vi "Functional Global - Raw Inputs and Outputs.vi"(7 "Functional Global Operation (Read)":T1=enum."Read", 10 "Outputs in":dbl[](array[numeric]), 11 "Inputs in":dbl[](array[numeric])) -> (2 "Outputs out":dbl[](array[numeric]), 3 "Inputs out":dbl[](array[numeric]))   [LabVIEW 2017]
uses:
  controls/Functional Global Operation.ctl
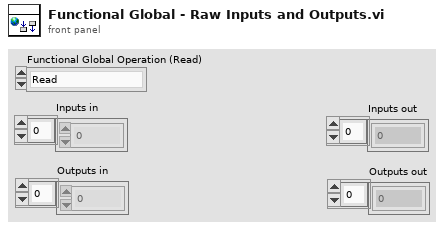
[diagram p1: front panel]
types:
  T1 = typedef "Functional Global Operation.ctl" = enum16{"Initialize", "Read", "Write"}
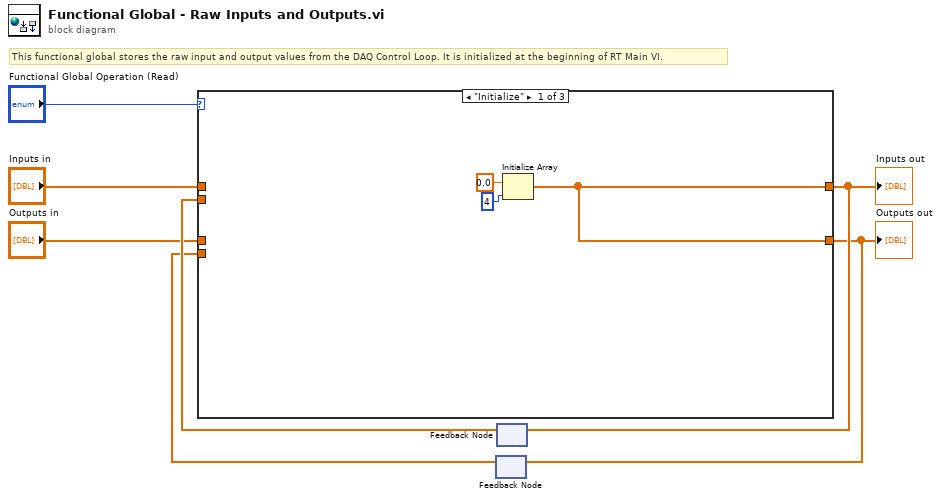
[diagram p0: block diagram]
diagram:
  # "This functional global stores the raw input and output values from the DAQ Control Loop. It is initialized at the beginning of RT Main VI."
  n1 = feedback #1() -> (w1:dbl[])  [unwired: 1 in]
  n2 = feedback #2() -> (w5:dbl[])  [unwired: 1 in]
  n3 = case shown="\"Initialize\"" "Functional Global Operation (Read)" {
    tunnel: "Inputs in" -> [_ _ w14]
    tunnel: [w8 w12 w14] -> w4
    tunnel: w5 -> [_ w12 _]
    tunnel: "Outputs in" -> [_ _ w13]
    tunnel: [w8 w11 w13] -> w2
    tunnel: w1 -> [_ w11 _]
    frame "Initialize" {
      n4 = Initialize Array(0.0 ("element"), 4 ("dimension size")) -> (w8:dbl[])
    }
    frame "Read", Default {
    }
    frame "Write" {
    }
  }
  "Inputs out" <- w4
  "Outputs out" <- w2
  n5 = feedback-in #1(w2) -> ()
  n6 = feedback-in #2(w4) -> ()
